vi "TTT_AI2.vi"() -> ()   [LabVIEW 2017]
uses:
  C:/Users/MohammadZahirul/Desktop/TicTacToe_Doc/Element 2.ctl
  Opponent.vi
panel:
  in  "Registerkarte":enum32{"spiel", "Start", "Begr."}(tab)
  in  "Boolesch 4":bool
  in  "Farbe2":T1 max=16777215 format="%6d"
  in  "Boolesch 3":bool
  in  "Boolesch 2":bool
  in  "Boolesch":bool
  out "Scoreboard":T2(tab)
  out "Score_L":T3
  out "Score_M":T3
  out "Score_U":T3
  out "Score_MF":T3
  out "Ausgabe":string
  out "Scoring":bool
  out "Toggle turn 2":bool
  in  "Toggle turn":bool
  in  "BoolArray":bool[][](array[boolean])
  out "Array":i8[][](array[ring])
  in  "Zeile x Spalte":i8=3 min=3 max=3
  in  "stop":bool
  in  "NewGame":bool
  out "ShowLed":bool
  out "Game Over":bool
  out "O Won":bool
  out "X Won":bool
  out "Next Turn":i8
  out "GewinnerRing":u16(ring)=1
  in  "Enum":T4(ring)
  in  "Farbe ändern":u32(colorbox)
  in  "Name":string
  in  "NameEinV":bool
  in  "Abbrechen":bool
  in  "EingabeBestätigung":bool
  out "AnzeigeBegrüß":string
  out "hidenArray":u8[][](array[numeric])
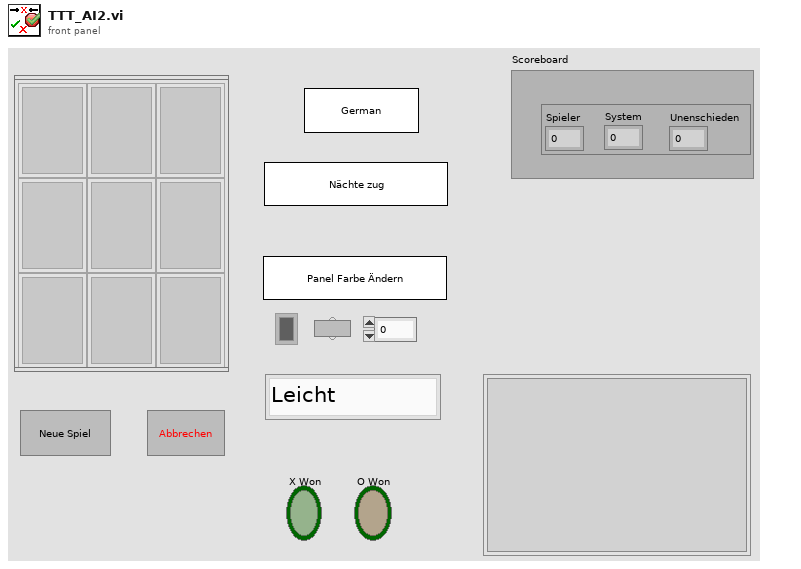
[diagram p1: front panel]
types:
  T1 = typedef "Element 2.ctl" = u32
  T2 = enum32{"Seite 1", "Seite 2", "Seite 3", "Seite 4"}
  T3 = cluster{"Spieler":u32, "System":u32, "Unenschieden":u32}
  T4 = enum16{"Leicht", "Mittel", "Unmöglich", "Mit einem Freund Spielen"}
  T5 = enum8{"Enabled", "Disabled", "Disabled and Grayed Out"}
  T6 = cluster{"Spieler":dbl, "Rechner":dbl, "Draw":dbl}
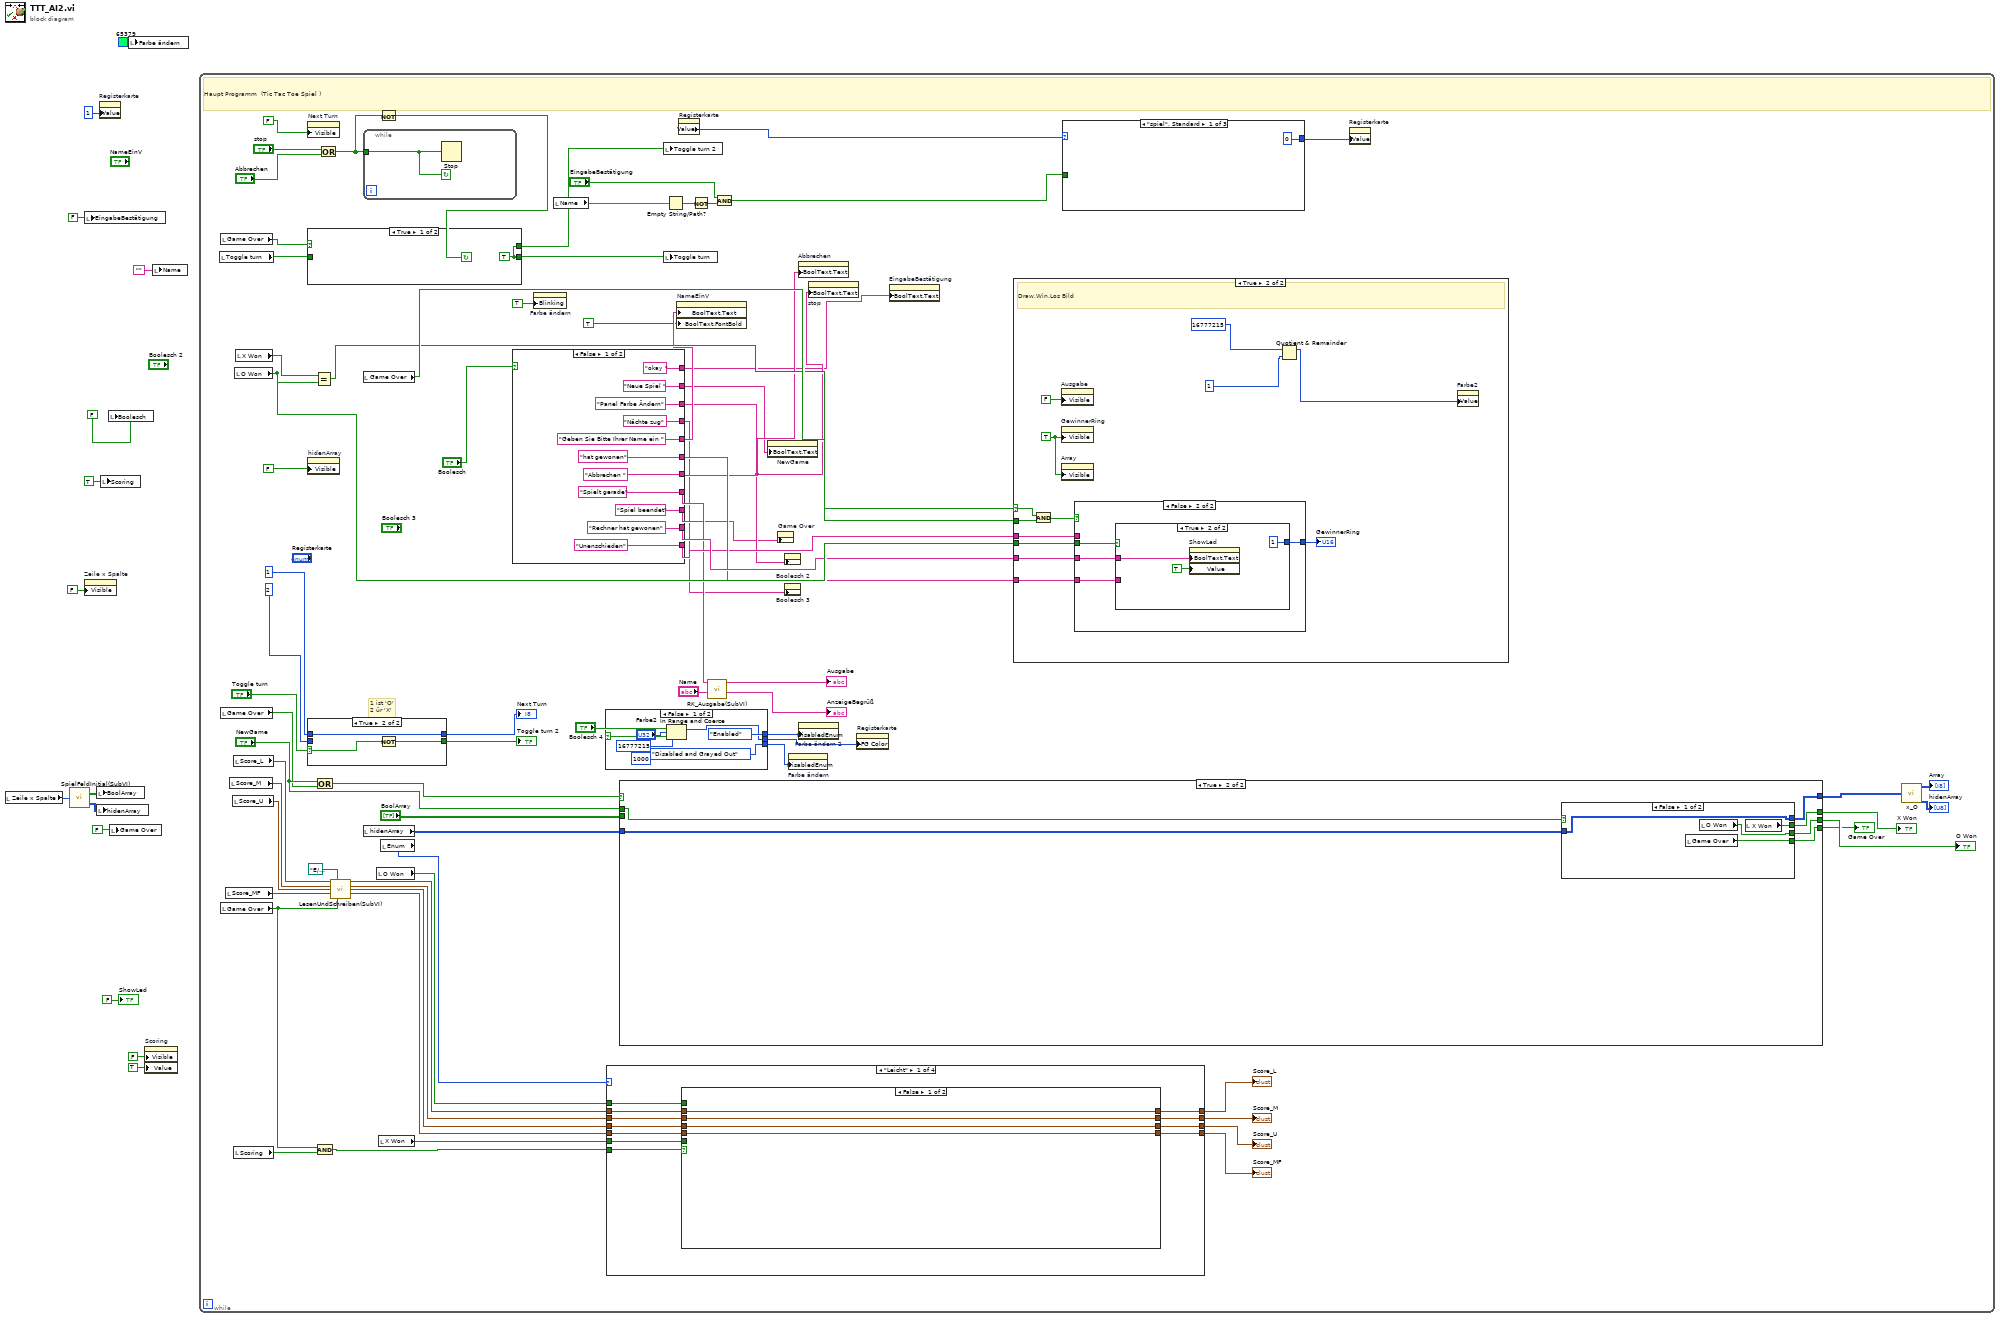
[diagram p0: block diagram]
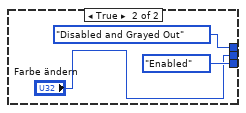
[diagram p2: hidden frame]
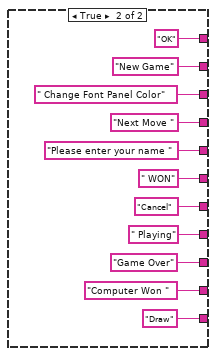
[diagram p3: hidden frame]
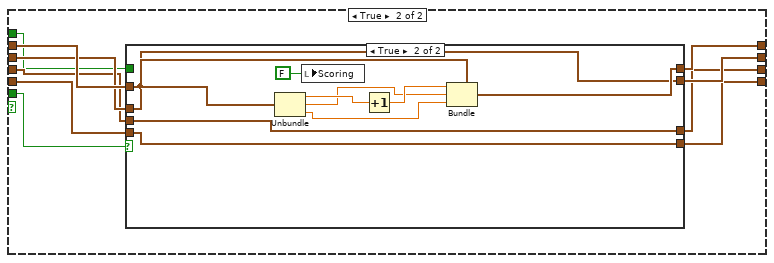
[diagram p4: hidden frame]
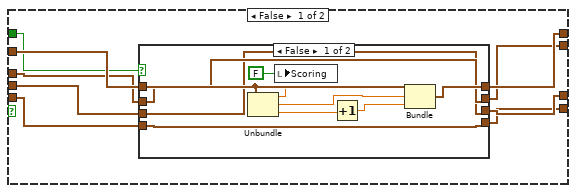
[diagram p5: hidden frame]
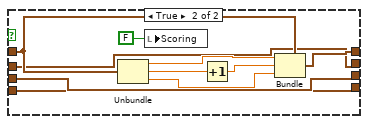
[diagram p6: hidden frame]
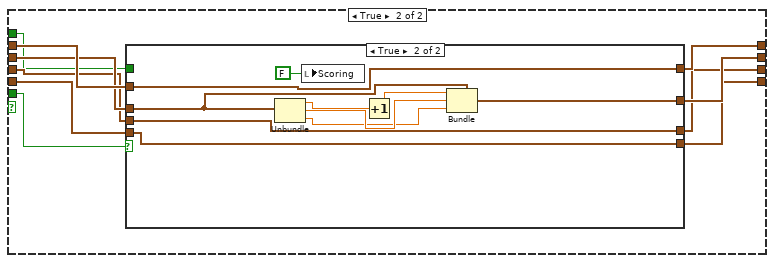
[diagram p8: hidden frame]
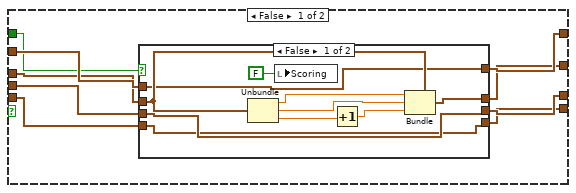
[diagram p9: hidden frame]
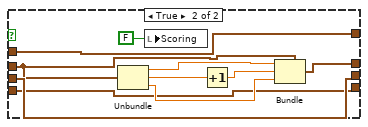
[diagram p10: hidden frame]
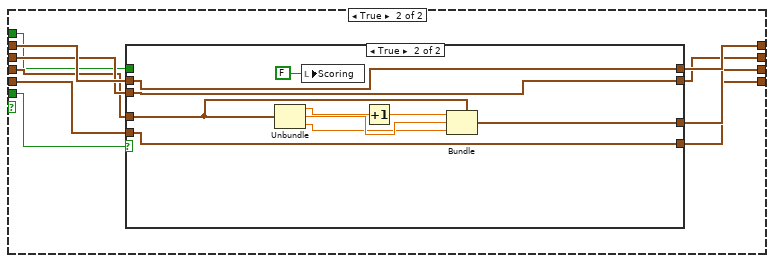
[diagram p12: hidden frame]
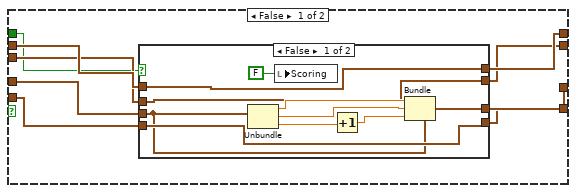
[diagram p13: hidden frame]
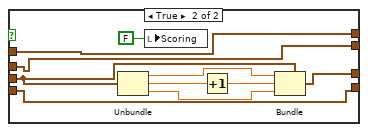
[diagram p14: hidden frame]
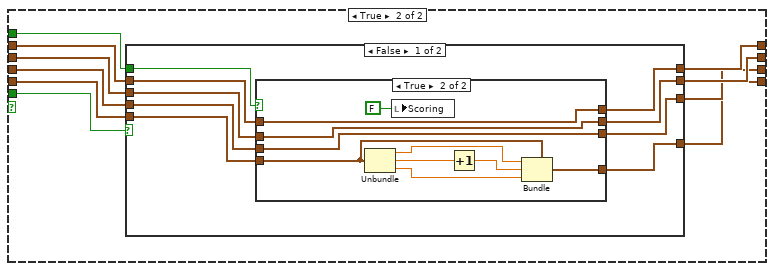
[diagram p16: hidden frame]
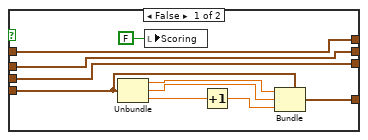
[diagram p17: hidden frame]
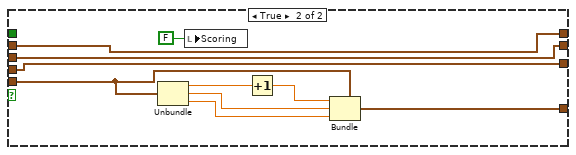
[diagram p18: hidden frame]
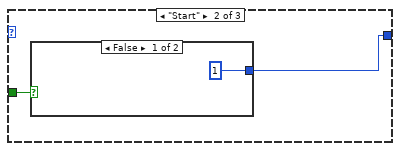
[diagram p19: hidden frame]
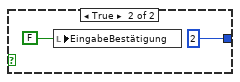
[diagram p20: hidden frame]
diagram:
  n1 = local read "Zeile x Spalte"() -> (w13:i8)
  n2 = call "SpielFeldInitial(SubVI).vi"("SpalteUndZeile"=w13) -> ("LEDArray"=w10:bool[][], "Grafikring"=w9:i8[][])
  n3 = property on="Zeile x Spalte" class="DigWert (strikt)"("Visible"=FALSE) -> ()  [unwired: 2 in, 2 out]
  n4 = local write "EingabeBestätigung"(FALSE) -> ()
  n5 = local write "BoolArray"(w10) -> ()
  n6 = local write "hidenArray"(w9) -> ()
  n7 = property on="Registerkarte" class="RKElem (strikt)"("Value"=1) -> ()  [unwired: 2 in, 2 out]
  n8 = local write "Scoring"(TRUE) -> ()
  n9 = local write "Boolesch"(FALSE) -> ()
  n10 = local write "Game Over"(FALSE) -> ()
  n11 = local write "Farbe ändern"(u32 65379 ("Panel Farbe")) -> ()
  n12 = property on="Scoring" class="Bool. (strikt)"("Visible"=FALSE, "Value"=TRUE) -> ()  [unwired: 2 in, 2 out]
  n13 = local write "Name"("") -> ()
  n14 = while {
    stop <- w54 continue-if-true
    # "1 ist 'O'\n2 ür 'X'"
    # "Haupt Programm  (Tic Tac Toe Spiel )"
    n15 = local read "Toggle turn"() -> (w79:bool)
    n16 = local read "Game Over"() -> (w64:bool)
    n17 = local read "Game Over"() -> (w71:bool)
    n18 = local read "Game Over"() -> (w33:bool)
    n19 = local read "Score_MF"() -> (w47:T3)
    n20 = local read "Score_M"() -> (w49:T3)
    n21 = local read "Score_U"() -> (w48:T3)
    n22 = local read "Score_L"() -> (w50:T3)
    n23 = local read "Scoring"() -> (w51:bool)
    n24 = local read "O Won"() -> (w74:bool)
    n25 = local read "X Won"() -> (w75:bool)
    n26 = property on="Next Turn" class="DigWert (strikt)"("Visible"=FALSE) -> ()  [unwired: 2 in, 2 out]
    n27 = case shown="True" w64 {
      tunnel: [w387 w389] -> w81
      tunnel: [w387 w388] -> w80
      tunnel: w79 -> [_ w389]
      frame True {
        w387 = TRUE
      }
      frame False {
        n28 = Not(x=w389) -> (.not. x?=w388:bool)
      }
    }
    n29 = property on="hidenArray" class="Array (strikt)"("Visible"=FALSE) -> ()  [unwired: 2 in, 2 out]
    n30 = case shown="True" "Toggle turn" {
      selector: "Toggle turn" -> [w424 w427]
      tunnel: 1 -> [_ w425]
      tunnel: 2 -> [w422 _]
      tunnel: [w422 w425] -> w89
      tunnel: [w423 w426] -> w82
      frame False {
        n31 = Not(x=w424) -> (.not. x?=w423:bool)
      }
      frame True {
        n32 = Not(x=w427) -> (.not. x?=w426:bool)
      }
    }
    "Next Turn" <- w89
    "Toggle turn 2" <- w82
    n33 = Equal?(x=w75, y=w74) -> (x = y?=w73:bool)
    n34 = Compound Arithmetic op=OR ("Mehrfacharithmetik")("NewGame", w71) -> (w88:bool)
    n35 = Compound Arithmetic op=AND ("Mehrfacharithmetik")(w33, w51) -> (w34:bool)
    n36 = Or(x="stop", y="Abbrechen") -> (x .or. y?=w55:bool)
    n37 = call "LesenUndSchreiben(SubVI).vi"("Score"=w50, "file path (dialog if empty)"=path "E:/Electrotechnik/Labview/praktikum/Ergebnis_TTT.txt", "Score 2"=w49, "Score 3"=w48, "Score 4"=w47, "gameOver"=w33) -> ("Score 5"=w46:T6, "Score 6"=w45:T6, "Score 7"=w44:T6, "Score 8"=w43:T6)  [unwired: 6 in]
    n38 = while {
      tunnel: w55 -> [w390]
      stop <- w390 continue-if-true
      n39 = Stop(stop? (T)=w390) -> ()
    }
    n40 = local read "Game Over"() -> (w76:bool)
    n41 = local read "hidenArray"() -> (w69:u8[][])
    n42 = local read "O Won"() -> (w40:bool)
    n43 = local read "X Won"() -> (w41:bool)
    n44 = Not(x=w55) -> (.not. x?=w54:bool)
    n45 = local read "Enum"() -> (w35:T4)
    n46 = case shown="False" "Boolesch" {
      tunnel: ["Rechner hat gewonen" ("Boolescher Text.Text") "Computer Won " ("Boolescher Text.Text")] -> w31
      tunnel: ["hat gewonen" ("Boolescher Text.Text") " WON" ("Boolescher Text.Text")] -> w30
      tunnel: ["Unenschieden" ("Boolescher Text.Text") "Draw" ("Boolescher Text.Text")] -> w29
      tunnel: ["Spielt gerade" ("Boolescher Text.Text") " Playing" ("Boolescher Text.Text")] -> w28
      tunnel: ["Geben Sie Bitte Ihrer Name ein " "Please enter your name "] -> w27
      tunnel: ["Abbrechen " "Cancel"] -> w25
      tunnel: ["okay " "OK"] -> w24
      tunnel: ["Neue Spiel " "New Game"] -> w23
      tunnel: ["Panel Farbe Ändern" " Change Font Panel Color" ("Boolescher Text.Text")] -> w22
      tunnel: ["Spiel beendet" "Game Over"] -> w21
      tunnel: ["Nächte zug" "Next Move "] -> w20
      frame False {
      }
      frame True {
      }
    }
    n47 = property on="Farbe ändern" class="Farbfeld"("Blinking"=TRUE) -> ()  [unwired: 2 in, 2 out]
    n48 = local read "Name"() -> (w62:string)
    n49 = case shown="False" "Boolesch 4" {
      tunnel: [T5."Disabled and Grayed Out" ("Deaktiviert") T5."Enabled" ("Deaktiviert")] -> w17
      tunnel: [T5."Enabled" ("Deaktiviert") T5."Disabled and Grayed Out" ("Deaktiviert")] -> w16
      tunnel: [w92 "Farbe ändern"] -> w15
      frame False {
        n50 = In Range and Coerce(upper limit=T1 16777215 ("Obergrenze"), x="Farbe2", lower limit=T1 1000 ("Untergrenze")) -> (coerced(x)=w92:T1)  [unwired: 1 out]
      }
      frame True {
      }
    }
    n51 = case shown="\"Leicht\"" w35 {
      tunnel: w34 -> [w133 w197 w261 w325]
      tunnel: w46 -> [w132 w196 w260 w324]
      tunnel: w45 -> [w131 w195 w259 w323]
      tunnel: w44 -> [w130 w194 w258 w322]
      tunnel: w43 -> [w129 w193 w257 w321]
      tunnel: w41 -> [w123 w192 w256 w315]
      tunnel: w40 -> [w128 w191 w255 w320]
      tunnel: [w127 w190 w254 w319] -> w39
      tunnel: [w126 w189 w253 w318] -> w38
      tunnel: [w125 w188 w252 w317] -> w37
      tunnel: [w124 w187 w251 w316] -> w36
      frame "Leicht" {
        n52 = case shown="False" w133 {
          tunnel: w132 -> [w137 w147]
          tunnel: w131 -> [w136 w145]
          tunnel: w130 -> [w135 w144]
          tunnel: w129 -> [w134 w143]
          tunnel: [w137 w146] -> w127
          tunnel: w128 -> [_ w142]
          tunnel: [w136 w141] -> w126
          tunnel: [w135 w138] -> w125
          tunnel: [w134 w140] -> w124
          tunnel: w123 -> [_ w139]
          frame False {
          }
          frame True {
            n53 = case shown="True" w139 {
              tunnel: w147 -> [w156 w181]
              tunnel: [w151 w186] -> w146
              tunnel: w145 -> [w155 w180]
              tunnel: w144 -> [w154 w179]
              tunnel: w143 -> [w153 w178]
              tunnel: w142 -> [w152 _]
              tunnel: [w150 w180] -> w141
              tunnel: [w149 w179] -> w138
              tunnel: [w148 w178] -> w140
              frame False {
                n54 = case shown="False" w152 {
                  tunnel: w156 -> [w164 w175]
                  tunnel: w155 -> [w160 w170]
                  tunnel: w154 -> [w159 w169]
                  tunnel: w153 -> [w158 w168]
                  tunnel: [w165 w171] -> w151
                  tunnel: [w160 w170] -> w150
                  tunnel: [w159 w169] -> w149
                  tunnel: [w158 w168] -> w148
                  frame False {
                    n55 = Unbundle(w164) -> ("Spieler"=w161:dbl, "Rechner"=w166:dbl, "Draw"=w163:dbl)
                    n56 = local write "Scoring"(FALSE) -> ()
                    n57 = Increment(x=w163) -> (x+1=w162:dbl)
                    n58 = Bundle(cluster=w164, "Spieler"=w161, "Rechner"=w166, "Draw"=w162) -> (w165:T6)
                  }
                  frame True {
                    n59 = Unbundle(w175) -> ("Spieler"=w173:dbl, "Rechner"=w172:dbl, "Draw"=w176:dbl)
                    n60 = local write "Scoring"(FALSE) -> ()
                    n61 = Increment(x=w172) -> (x+1=w174:dbl)
                    n62 = Bundle(cluster=w175, "Spieler"=w173, "Rechner"=w174, "Draw"=w176) -> (w171:T6)
                  }
                }
              }
              frame True {
                n63 = Unbundle(w181) -> ("Spieler"=w185:dbl, "Rechner"=w183:dbl, "Draw"=w182:dbl)
                n64 = local write "Scoring"(FALSE) -> ()
                n65 = Increment(x=w185) -> (x+1=w184:dbl)
                n66 = Bundle(cluster=w181, "Spieler"=w184, "Rechner"=w183, "Draw"=w182) -> (w186:T6)
              }
            }
          }
        }
      }
      frame "Mittel" {
        n67 = case shown="False" w197 {
          tunnel: w196 -> [w201 w211]
          tunnel: w195 -> [w200 w209]
          tunnel: w194 -> [w199 w208]
          tunnel: w193 -> [w198 w207]
          tunnel: [w201 w210] -> w190
          tunnel: w192 -> [_ w206]
          tunnel: w191 -> [_ w205]
          tunnel: [w200 w204] -> w189
          tunnel: [w199 w203] -> w188
          tunnel: [w198 w202] -> w187
          frame False {
          }
          frame True {
            n68 = case shown="True" w206 {
              tunnel: w211 -> [w220 w242]
              tunnel: [w215 w242] -> w210
              tunnel: w209 -> [w219 w244]
              tunnel: w208 -> [w218 w246]
              tunnel: w207 -> [w217 w245]
              tunnel: w205 -> [w216 _]
              tunnel: [w214 w243] -> w204
              tunnel: [w213 w246] -> w203
              tunnel: [w212 w245] -> w202
              frame False {
                n69 = case shown="False" w216 {
                  tunnel: w220 -> [w222 w232]
                  tunnel: w219 -> [w223 w234]
                  tunnel: w218 -> [w226 w236]
                  tunnel: w217 -> [w225 w235]
                  tunnel: [w222 w232] -> w215
                  tunnel: [w224 w233] -> w214
                  tunnel: [w226 w236] -> w213
                  tunnel: [w225 w235] -> w212
                  frame False {
                    n70 = Unbundle(w223) -> ("Spieler"=w227:dbl, "Rechner"=w230:dbl, "Draw"=w229:dbl)
                    n71 = local write "Scoring"(FALSE) -> ()
                    n72 = Increment(x=w229) -> (x+1=w228:dbl)
                    n73 = Bundle(cluster=w223, "Spieler"=w227, "Rechner"=w230, "Draw"=w228) -> (w224:T6)
                  }
                  frame True {
                    n74 = Unbundle(w234) -> ("Spieler"=w238:dbl, "Rechner"=w237:dbl, "Draw"=w240:dbl)
                    n75 = local write "Scoring"(FALSE) -> ()
                    n76 = Increment(x=w237) -> (x+1=w239:dbl)
                    n77 = Bundle(cluster=w234, "Spieler"=w238, "Rechner"=w239, "Draw"=w240) -> (w233:T6)
                  }
                }
              }
              frame True {
                n78 = Unbundle(w244) -> ("Spieler"=w250:dbl, "Rechner"=w248:dbl, "Draw"=w247:dbl)
                n79 = local write "Scoring"(FALSE) -> ()
                n80 = Increment(x=w250) -> (x+1=w249:dbl)
                n81 = Bundle(cluster=w244, "Spieler"=w249, "Rechner"=w248, "Draw"=w247) -> (w243:T6)
              }
            }
          }
        }
      }
      frame "Unmöglich" {
        n82 = case shown="False" w261 {
          tunnel: w260 -> [w262 w275]
          tunnel: w259 -> [w265 w273]
          tunnel: w258 -> [w264 w272]
          tunnel: w257 -> [w263 w271]
          tunnel: [w262 w274] -> w254
          tunnel: w256 -> [_ w270]
          tunnel: w255 -> [_ w269]
          tunnel: [w265 w268] -> w253
          tunnel: [w264 w267] -> w252
          tunnel: [w263 w266] -> w251
          frame False {
          }
          frame True {
            n83 = case shown="True" w270 {
              tunnel: w275 -> [w284 w306]
              tunnel: [w279 w306] -> w274
              tunnel: w273 -> [w283 w310]
              tunnel: w272 -> [w282 w308]
              tunnel: w271 -> [w281 w309]
              tunnel: w269 -> [w280 _]
              tunnel: [w278 w310] -> w268
              tunnel: [w277 w307] -> w267
              tunnel: [w276 w309] -> w266
              frame False {
                n84 = case shown="False" w280 {
                  tunnel: w284 -> [w286 w296]
                  tunnel: w283 -> [w290 w300]
                  tunnel: w282 -> [w287 w297]
                  tunnel: w281 -> [w289 w299]
                  tunnel: [w286 w296] -> w279
                  tunnel: [w290 w300] -> w278
                  tunnel: [w288 w298] -> w277
                  tunnel: [w289 w299] -> w276
                  frame False {
                    n85 = Unbundle(w287) -> ("Spieler"=w291:dbl, "Rechner"=w294:dbl, "Draw"=w293:dbl)
                    n86 = local write "Scoring"(FALSE) -> ()
                    n87 = Increment(x=w293) -> (x+1=w292:dbl)
                    n88 = Bundle(cluster=w287, "Spieler"=w291, "Rechner"=w294, "Draw"=w292) -> (w288:T6)
                  }
                  frame True {
                    n89 = Unbundle(w297) -> ("Spieler"=w302:dbl, "Rechner"=w301:dbl, "Draw"=w304:dbl)
                    n90 = local write "Scoring"(FALSE) -> ()
                    n91 = Increment(x=w301) -> (x+1=w303:dbl)
                    n92 = Bundle(cluster=w297, "Spieler"=w302, "Rechner"=w303, "Draw"=w304) -> (w298:T6)
                  }
                }
              }
              frame True {
                n93 = Unbundle(w308) -> ("Spieler"=w314:dbl, "Rechner"=w312:dbl, "Draw"=w311:dbl)
                n94 = local write "Scoring"(FALSE) -> ()
                n95 = Increment(x=w314) -> (x+1=w313:dbl)
                n96 = Bundle(cluster=w308, "Spieler"=w313, "Rechner"=w312, "Draw"=w311) -> (w307:T6)
              }
            }
          }
        }
      }
      frame "Mit einem Freund Spielen" {
        n97 = case shown="False" w325 {
          tunnel: w324 -> [w329 w339]
          tunnel: w323 -> [w328 w337]
          tunnel: w322 -> [w327 w336]
          tunnel: w321 -> [w326 w335]
          tunnel: [w329 w338] -> w319
          tunnel: w320 -> [_ w334]
          tunnel: [w328 w333] -> w318
          tunnel: [w327 w332] -> w317
          tunnel: [w326 w331] -> w316
          tunnel: w315 -> [_ w330]
          frame False {
          }
          frame True {
            n98 = case shown="False" w330 {
              tunnel: w339 -> [w348 w372]
              tunnel: [w343 w372] -> w338
              tunnel: w337 -> [w347 w374]
              tunnel: w336 -> [w346 w371]
              tunnel: w335 -> [w345 w373]
              tunnel: w334 -> [w344 _]
              tunnel: [w342 w374] -> w333
              tunnel: [w341 w371] -> w332
              tunnel: [w340 w370] -> w331
              frame False {
                n99 = case shown="True" w344 {
                  tunnel: w348 -> [w350 w360]
                  tunnel: w347 -> [w354 w364]
                  tunnel: w346 -> [w353 w363]
                  tunnel: w345 -> [w352 w362]
                  tunnel: [w350 w360] -> w343
                  tunnel: [w354 w364] -> w342
                  tunnel: [w353 w363] -> w341
                  tunnel: [w351 w361] -> w340
                  frame False {
                    n100 = Unbundle(w352) -> ("Spieler"=w355:dbl, "Rechner"=w358:dbl, "Draw"=w357:dbl)
                    n101 = local write "Scoring"(FALSE) -> ()
                    n102 = Increment(x=w357) -> (x+1=w356:dbl)
                    n103 = Bundle(cluster=w352, "Spieler"=w355, "Rechner"=w358, "Draw"=w356) -> (w351:T6)
                  }
                  frame True {
                    n104 = Unbundle(w362) -> ("Spieler"=w366:dbl, "Rechner"=w365:dbl, "Draw"=w368:dbl)
                    n105 = local write "Scoring"(FALSE) -> ()
                    n106 = Increment(x=w365) -> (x+1=w367:dbl)
                    n107 = Bundle(cluster=w362, "Spieler"=w366, "Rechner"=w367, "Draw"=w368) -> (w361:T6)
                  }
                }
              }
              frame True {
                n108 = Unbundle(w373) -> ("Spieler"=w378:dbl, "Rechner"=w376:dbl, "Draw"=w375:dbl)
                n109 = local write "Scoring"(FALSE) -> ()
                n110 = Increment(x=w378) -> (x+1=w377:dbl)
                n111 = Bundle(cluster=w373, "Spieler"=w377, "Rechner"=w376, "Draw"=w375) -> (w370:T6)
              }
            }
          }
        }
      }
    }
    "Score_L" <- w39
    "Score_M" <- w38
    "Score_U" <- w37
    "Score_MF" <- w36
    n112 = case shown="True" w88 {
      tunnel: [w436 w535] -> w86
      tunnel: "BoolArray" -> [w438 _]
      tunnel: [w437 w534] -> w85
      tunnel: "NewGame" -> [_ w531]
      tunnel: w69 -> [w435 w532]
      tunnel: [w429 w533] -> w67
      tunnel: [w430 w530] -> w77
      frame False {
        n113 = local read "Next Turn"() -> (w434:i8)
        n114 = case shown="1, Standard" w434 {
          selector: w434 -> [w443 w500]
          tunnel: w438 -> [w444 w501]
          tunnel: w435 -> [w442 w502]
          tunnel: [w441 w499] -> w429
          tunnel: "Enum" -> [w440 _]
          frame 1, Default {
            n115 = case shown="\"Unmöglich\"" w440 {
              tunnel: w444 -> [w454 w460 w470 w477]
              tunnel: w443 -> [w451 w459 w466 w476]
              tunnel: w442 -> [w455 w461 w468 w475]
              tunnel: [w449 w464 w467 w474] -> w441
              tunnel: [2 0 1 3] -> w439
              frame "Unmöglich" {
                # "Minimax Algorithmen"
                n116 = call "Minimax.vi"("Game"=w455, "Active Turn"=w451, "NextTurn"=w451) -> ("Next Move"=w456:cluster{"Row":i32, "Col":i32})  [unwired: 13 in, 3 out]
                n117 = Unbundle(w456) -> ("Row"=w453:i32, "Col"=w452:i32)
                n118 = local read "Toggle turn"() -> (w447:bool)
                n119 = Replace Array Subset(array=w455, new element=w451, index (row)=w453, index (col)=w452) -> (w449:u8[][])
                n120 = Replace Array Subset(array=w454, new element=TRUE, index (row)=w453, index (col)=w452) -> (w448:bool[][])
                n121 = local write "BoolArray"(w448) -> ()
                n122 = Not(x=w447) -> (.not. x?=w446:bool)
                n123 = local write "Toggle turn"(w446) -> ()
              }
              frame "Leicht" {
                # "Simple strategie"
                n124 = local read "Toggle turn"() -> (w458:bool)
                n125 = call "SimpelStrategie(SubVI).vi"("toggle"=w458, "NextTurn"=w459, "BoolArray"=w460, "Array"=w461) -> ("toggle 2"=w462:bool, "Array 3"=w463:bool[][], "Array 2"=w464:u8[][])  [unwired: 1 in]
                n126 = local write "BoolArray"(w463) -> ()
                n127 = local write "Toggle turn"(w462) -> ()
              }
              frame "Mittel", Default {
                # "SubVi mit Zufall Zahl Strategie"
                n128 = local read "Toggle turn"() -> (w471:bool)
                n129 = call "ZufallFeldGenarator (SubVI).vi"("Numerisch"=w466, "BoolArray (Eingang)"=w470, "Tic Tac Toe (Eingang)"=w468, "Toggle turn (Eingang)"=w471) -> ("BoolArray (Ausgang)"=w469:bool[][], "Tic Tac Toe (Ausgang)"=w467:u8[][], "Toggle turn (Ausgang)"=w472:bool)  [unwired: 1 in]
                n130 = local write "Toggle turn"(w472) -> ()
                n131 = local write "BoolArray"(w469) -> ()
              }
              frame "Mit einem Freund Spielen" {
                n132 = for {
                  tunnel: w477 -> [w481] mode=indexing
                  tunnel: w476 -> [w480]
                  tunnel: w475 -> [w479] mode=indexing
                  tunnel: [w478] -> w474 mode=indexing
                  n133 = for {
                    tunnel: w481 -> [w490] mode=indexing
                    tunnel: w480 -> [w482]
                    tunnel: w479 -> [w484] mode=indexing
                    tunnel: [w483] -> w478 mode=indexing
                    n134 = Not Equal?(x=w484, y=1) -> (x != y?=w493:bool)
                    n135 = Not Equal?(x=2, y=w484) -> (x != y?=w492:bool)
                    n136 = And(x=w493, y=w492) -> (x .and. y?=w491:bool)
                    n137 = local read "Toggle turn"() -> (w487:bool)
                    n138 = And(x=w490, y=w491) -> (x .and. y?=w489:bool)
                    n139 = case shown="True" w489 {
                      tunnel: [w495 w498] -> w488
                      tunnel: w487 -> [w495 w497]
                      tunnel: [w494 w496] -> w483
                      tunnel: w484 -> [w494 _]
                      tunnel: w482 -> [_ w496]
                      frame False {
                      }
                      frame True {
                        n140 = Not(x=w497) -> (.not. x?=w498:bool)
                      }
                    }
                    n141 = local write "Toggle turn"(w488) -> ()
                  }
                }
              }
            }
            "Scoreboard" <- w439
          }
          frame 2 {
            n142 = for {
              tunnel: w502 -> [w506] mode=indexing
              tunnel: w501 -> [w505] mode=indexing
              tunnel: w500 -> [w504]
              tunnel: [w503] -> w499 mode=indexing
              n143 = for {
                tunnel: w506 -> [w509] mode=indexing
                tunnel: w505 -> [w513] mode=indexing
                tunnel: w504 -> [w511]
                tunnel: [w510] -> w503 mode=indexing
                n144 = Not Equal?(x=w509, y=u8 1) -> (x != y?=w516:bool)
                n145 = Not Equal?(x=w509, y=u8 2) -> (x != y?=w515:bool)
                n146 = And(x=w516, y=w515) -> (x .and. y?=w514:bool)
                n147 = local read "Toggle turn"() -> (w508:bool)
                n148 = And(x=w514, y=w513) -> (x .and. y?=w512:bool)
                n149 = case shown="False" w512 {
                  tunnel: w511 -> [_ w523]
                  tunnel: [w520 w523] -> w510
                  tunnel: w509 -> [w520 _]
                  tunnel: w508 -> [w519 w521]
                  tunnel: [w519 w522] -> w507
                  frame False {
                  }
                  frame True {
                    n150 = Not(x=w521) -> (.not. x?=w522:bool)
                  }
                }
                n151 = local write "Toggle turn"(w507) -> ()
              }
            }
          }
        }
        n152 = local read "Next Turn"() -> (w428:i8)
        n153 = call "Score.vi"("Turn Taking Player"=w428, "Game"=w429) -> ("Game over"=w431:bool, "Win"=w432:bool)  [unwired: 7 in, 1 out]
        n154 = case shown="1, Standard" w428 {
          tunnel: [FALSE w529] -> w437
          tunnel: w432 -> [w525 w529]
          tunnel: [w525 FALSE] -> w436
          tunnel: w431 -> [w524 w527]
          tunnel: [w524 w527] -> w430
          frame 2 {
            # "Hier wird \nwin_check\n weiter sortiert \nnach Spieler"
          }
          frame 1, Default {
          }
        }
      }
      frame True {
        n155 = case shown="False" w531 {
          tunnel: [w538 w544] -> w535
          tunnel: [w539 w544] -> w534
          tunnel: [w537 w541] -> w533
          tunnel: w532 -> [w537 _]
          tunnel: [w536 w544] -> w530
          frame False {
            n156 = local read "Game Over"() -> (w536:bool)
            n157 = local read "O Won"() -> (w539:bool)
            n158 = local read "X Won"() -> (w538:bool)
          }
          frame True {
            w544 = FALSE
            n159 = call "SpielFeldInitial(SubVI).vi"("SpalteUndZeile"="Zeile x Spalte") -> ("LEDArray"=w542:bool[][], "Grafikring"=w541:i8[][])
            n160 = local write "BoolArray"(w542) -> ()
            "Scoring" <- TRUE
          }
        }
      }
    }
    "X Won" <- w86
    "O Won" <- w85
    "Game Over" <- w77
    n161 = local write "Toggle turn 2"(w80) -> ()
    n162 = local write "Toggle turn"(w81) -> ()
    n163 = Empty String/Path?(string/path=w62) -> (empty?=w61:bool)
    n164 = property on="NameEinV" class="Bool."("BoolText.Text"=w27, "BoolText.FontBold"=TRUE ("Boolescher Text.Schriftart:Fett")) -> ()  [unwired: 2 in, 2 out]
    n165 = property on="Registerkarte" class="RKElem (strikt)"() -> ("Value"=w63:enum32{"spiel", "Start", "Begr."})  [unwired: 2 in, 2 out]
    n166 = Not(x=w61) -> (.not. x?=w52:bool)
    n167 = call "RK_Ausgabe(SubVI).vi"("Name"="Name", "werS"=w28) -> ("AnzeigeBegrüß"=→"AnzeigeBegrüß":string, "AnzeigeOben"=→"Ausgabe":string)  [unwired: 8 in]
    n168 = Compound Arithmetic op=AND ("Mehrfacharithmetik")("EingabeBestätigung", w52) -> (w59:bool)
    n169 = property on="NewGame" class="Bool."("BoolText.Text"=w23) -> ()  [unwired: 2 in, 2 out]
    n170 = property on="Game Over" class="Bool. (strikt)"("BoolText.Text"=w21) -> ()  [unwired: 2 in, 2 out]
    n171 = property on="Boolesch 2" class="Bool."("BoolText.Text"=w22) -> ()  [unwired: 2 in, 2 out]
    n172 = property on="Boolesch 3" class="Bool."("BoolText.Text"=w20) -> ()  [unwired: 2 in, 2 out]
    n173 = property on="Farbe ändern" class="Farbfeld"("DisabledEnum"=w17) -> ()  [unwired: 2 in, 2 out]
    n174 = property on="Abbrechen" class="Bool."("BoolText.Text"=w25) -> ()  [unwired: 2 in, 2 out]
    n175 = property on="Farbe ändern 2" class="DigWert (strikt)"("DisabledEnum"=w16) -> ()  [unwired: 2 in, 2 out]
    n176 = property on="stop" class="Bool."("BoolText.Text"=w25) -> ()  [unwired: 2 in, 2 out]
    n177 = property on="Registerkarte" class="RKElem (strikt)"("FG Color"=w15) -> ()  [unwired: 2 in, 2 out]
    n178 = property on="EingabeBestätigung" class="Bool. (strikt)"("BoolText.Text"=w24) -> ()  [unwired: 2 in, 2 out]
    n179 = case shown="True" w76 {
      selector: w76 -> [_ w397]
      tunnel: w74 -> [_ w404]
      tunnel: w73 -> [_ w403]
      tunnel: w31 -> [_ w401]
      tunnel: w30 -> [_ w400]
      tunnel: w29 -> [_ w399]
      frame False {
        w392 = FALSE
        w391 = TRUE ("Sichtbar")
        # "wenn das Spiel nicht beendet !"
        n180 = property on="ShowLed" class="Bool. (strikt)"("BoolText.Text"="" ("Boolescher Text.Text"), "Value"=w392) -> ()  [unwired: 2 in, 2 out]
        n181 = property on="Ausgabe" class="Str"("Visible"=w391) -> ()  [unwired: 2 in, 2 out]
        n182 = property on="BoolArray" class="Arr"("Visible"=w391) -> ()  [unwired: 2 in, 2 out]
        n183 = property on="GewinnerRing" class="Ring (strikt)"("Visible"=w392) -> ()  [unwired: 2 in, 2 out]
      }
      frame True {
        w405 = TRUE ("Sichtbar")
        # "Draw,Win,Los Bild"
        n184 = And(x=w397, y=w403) -> (x .and. y?=w398:bool)
        n185 = property on="Ausgabe" class="Str"("Visible"=FALSE) -> ()  [unwired: 2 in, 2 out]
        n186 = property on="GewinnerRing" class="Ring (strikt)"("Visible"=w405) -> ()  [unwired: 2 in, 2 out]
        n187 = property on="Array" class="Arr (strikt)"("Visible"=w405) -> ()  [unwired: 2 in, 2 out]
        n188 = case shown="False" w398 {
          tunnel: [0 w412] -> w406
          tunnel: w404 -> [_ w413]
          tunnel: w401 -> [_ w411]
          tunnel: w400 -> [_ w410]
          tunnel: w399 -> [w407 _]
          frame True {
            n189 = property on="ShowLed" class="Bool. (strikt)"("BoolText.Text"=w407, "Value"=TRUE) -> ()  [unwired: 2 in, 2 out]
          }
          frame False {
            n190 = case shown="True" w413 {
              tunnel: [2 1] -> w412
              tunnel: w411 -> [_ w419]
              tunnel: w410 -> [w414 _]
              frame False {
                n191 = local read "Name"() -> (w416:string)
                n192 = Concatenate Strings(w416, w414) -> (w415:string)
                n193 = property on="ShowLed" class="Bool. (strikt)"("BoolText.Text"=w415, "Value"=TRUE) -> ()  [unwired: 2 in, 2 out]
              }
              frame True {
                n194 = property on="ShowLed" class="Bool. (strikt)"("BoolText.Text"=w419, "Value"=TRUE) -> ()  [unwired: 2 in, 2 out]
              }
            }
          }
        }
        "GewinnerRing" <- w406
        n195 = Quotient & Remainder(x=16777215, y=1) -> (x-y*floor(x/y)=w394:i32)  [unwired: 1 out]
        n196 = property on="Farbe2" class="DigWert (strikt)"("Value"=w394) -> ()  [unwired: 2 in, 2 out]
      }
    }
    n197 = case shown="\"spiel\", Standard" w63 {
      tunnel: [0 w381 0] -> w58
      tunnel: w59 -> [_ w380 _]
      frame "spiel", Default {
      }
      frame "Start" {
        n198 = case shown="False" w380 {
          tunnel: [1 2] -> w381
          frame False {
          }
          frame True {
            n199 = local write "EingabeBestätigung"(FALSE) -> ()
          }
        }
      }
      frame "Begr." {
        n200 = Wait Until Next ms Multiple(millisecond multiple=u32 1000 ("ms")) -> ()  [unwired: 1 out]
      }
    }
    n201 = property on="Registerkarte" class="RKElem (strikt)"("Value"=w58) -> ()  [unwired: 2 in, 2 out]
    n202 = call "x_O.vi"("Tic Tac Toe"=w67) -> ("GrafikRing"=→"Array":i32[][], "Game"=→"hidenArray":i32[][])  [unwired: 8 in]
  }
  "ShowLed" <- FALSE
